vi "LocalMemTrigger.vi"(6 "Channels":i32 format="%x", 8 "error in (no error)":errorcluster, 9 "Size":i32, 10 "Type":enum16{"ADC", "DAC"}(ring), 11 "RFSoC Driver in":refnum<class "RFSoC Driver.lvclass">) -> (0 "error out":errorcluster, 3 "RFSoC Driver out":refnum<class "RFSoC Driver.lvclass">)   [LabVIEW 2019, in "RFSoC Driver.lvclass"]
uses:
  RFSoC Driver.lvclass
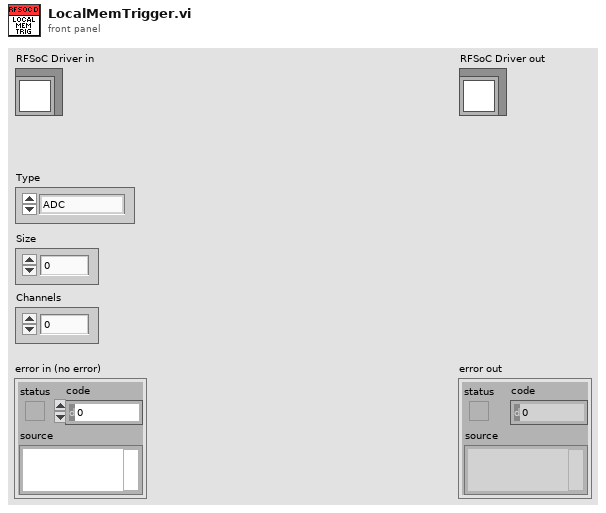
[diagram p1: front panel]
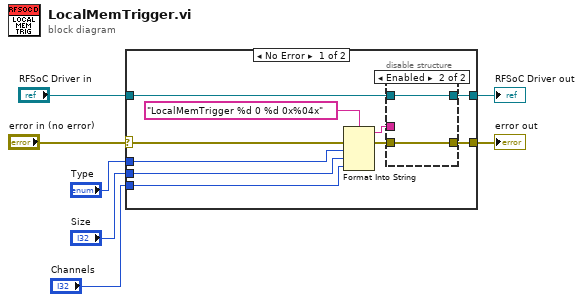
[diagram p0: block diagram]
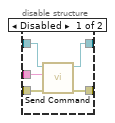
[diagram p2: hidden frame]
diagram:
  n1 = case shown="No Error" "error in (no error)" {
    selector: "error in (no error)" -> [w11 w26]
    tunnel: [w15 w26] -> w6
    tunnel: [w17 w25] -> w4
    tunnel: "RFSoC Driver in" -> [w16 w25]
    tunnel: "Type" -> [w13 _]
    tunnel: "Size" -> [w9 _]
    tunnel: "Channels" -> [w8 _]
    frame No Error {
      n2 = Format Into String(format string="LocalMemTrigger %d 0 %d 0x%04x", error in=w11, w13, w9, w8) -> (resulting string=w10:string, error out=w12:errorcluster)  [unwired: 1 in]
      n3 = disable-structure shown="Enabled" {
        disable-tunnel: [w22 w24] -> w17
        disable-tunnel: w16 -> [w21 w24]
        disable-tunnel: [w20 w23] -> w15
        disable-tunnel: w12 -> [w19 w23]
        disable-tunnel: w10 -> [w18 _]
        frame Disabled {
          n4 = call-dynamic "Send Command.vi"("error in (no error)"=w19, "Command"=w18, "RFSoC Driver in"=w21) -> ("error out"=w20:errorcluster, "RFSoC Driver out"=w22:refnum<class "RFSoC Driver.lvclass">)  [unwired: 6 in, 1 out]
        }
        frame Enabled {
        }
      }
    }
    frame Error {
    }
  }
  "error out" <- w6
  "RFSoC Driver out" <- w4
